vi "RPi HMI Loop.vi"() -> ()   [LabVIEW 2019]
uses:
  Controls/RPi HMI Mode.ctl
  Controls/HMI Global Mode.ctl
panel:
  in  "Power Relay":T1
  in  "Manual\nCMD":dbl[](array[numeric])=[0.0, 0.0, 0.0, 0.0, 0.0, 0.0] min=0.0 max=100.0 step=0.1 format="%#.2f"
  in  "Power Supply Cmd (V):":dbl min=0.0 max=20.0 format="%#.2f"
  in  "PressureCMD":dbl caption="Pressure Cmd (kPa):" min=0.0 max=825.0 format="%#.2f"
  in  "pb.Run Profile":bool
  in  "Tank 1 Setpoint":dbl caption="deg C"
  in  "Tank 2 Setpoint":dbl caption="deg C"
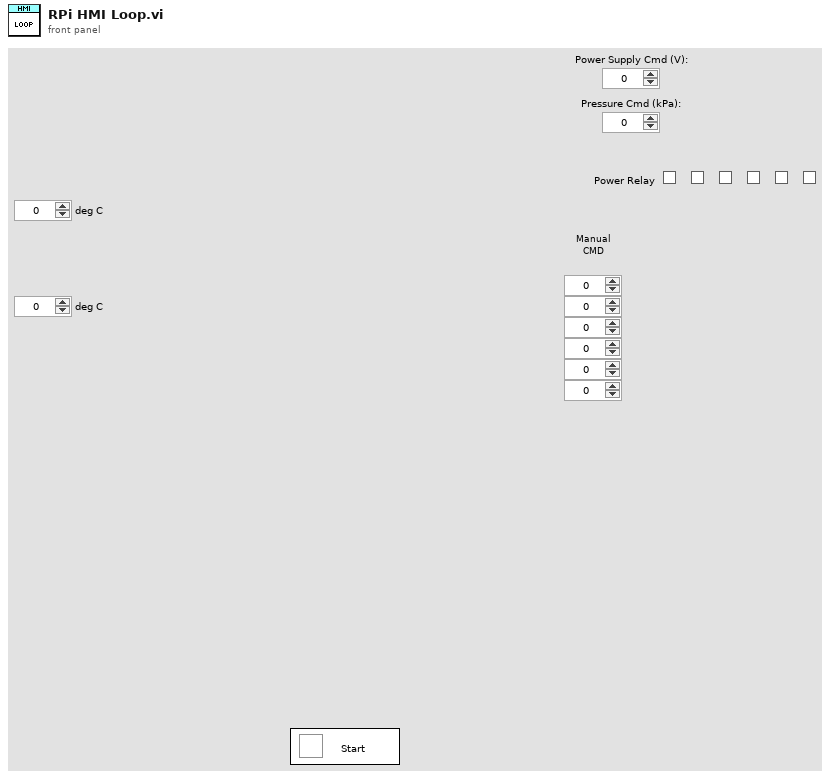
[diagram p1: front panel]
types:
  T1 = cluster{"Pump 1":bool, "Pump 2":bool, "Pump 3":bool, "Pump 4":bool, "Pump 5":bool, "Pump 6":bool}
  T2 = typedef "RPi HMI Mode.ctl" = enum16{"Init", "Write Data", "Read from RPi", "Write to RPi", "Read HMI Cluster"}
  T3 = typedef "HMI Cluster.ctl" = cluster{"Error":errorcluster, "COM Ref":refnum<visa-resource-name>, "Pump Data":T4, "Tank Data":cluster{"PS Actual (V):":dbl, "Temp1":dbl, "Temp2":dbl}, "Power Relays":cluster{"Pump 1":bool, "Pump 2":bool, "Pump 3":bool, "Pump 4":bool, "Pump 5":bool, "Pump 6":bool}, "Pump CMDs":dbl[], "HMI Header":T5, "Tank CMDs":T6, "HMI Tog Buttons":T7, "In Test":bool, "HMI Command":bool, "HMI Mom Buttons":T8, "Controller Config":T9, "Alarm":bool, "Alarm Message 1":string, "Alarm Message 2":string, "Recording":bool, "Serial Numbers":string[], "Pumps Present":bool[]}
  T4 = typedef "Pump Data.ctl" = cluster{"Voltages":dbl[], "PumpCurrent":dbl[], "Speed":dbl[], "ControllerCurrent":dbl[], "Pressure":dbl[], "Flow":dbl[], "Elapsed Time (Display)":dbl[], "Avg Pressure":dbl, "Avg Speed":dbl, "Elapsed Time":dbl[], "Diagnostic":dbl[]}
  T5 = typedef "HMI Header.ctl" = cluster{"Line 1":string, "Line 2":string, "Line 3":string, "Line 4":string}
  T6 = typedef "Tank CMDs.ctl" = cluster{"PS CMD":dbl, "Press CMD":dbl, "Temp 1 CMD":dbl, "Temp 2 CMD":dbl, "AO2 CMD":dbl}
  T7 = typedef "HMI Tog Buttons.ctl" = cluster{"Start Test":bool, "Toggle Spare 1":bool, "Toggle Spare 2":bool, "Toggle Spare 3":bool, "Toggle Spare 4":bool, "Toggle Spare 5":bool}
  T8 = typedef "HMI Mom Buttons.ctl" = cluster{"Stop":bool, "Reset Timers":bool, "Log Fuel Change":bool, "Alarm Dismiss":bool}
  T9 = typedef "Controller Config.ctl" = cluster{"Controller Name":T10, "CommSeg":i32, "PWM?":bool, "Frequency":i32, "Low Command":dbl, "High Command":dbl, "Stop Command":dbl, "Command Step":dbl, "Solenoid Stop?":bool, "Controller?":bool, "Invert PWM":bool, "Flange Mount Ctrl":bool, "Diagnostic Mode":T11}
  T10 = typedef "Controller Names.ctl" = enum16{"Kuhnke", "Helbako BLDC", "Conti", "Hella BLDC OL PWM", "Hella BLDC Turbine OL PWM", "Hella BLDC Pressure", "Helbako (old)", "TI PWM", "PSA", "Hella Gas", "Hella Diesel", "8 Comm", "10 Comm", "8 Comm Hella", "10 Comm Hella", "8 Comm Omron", "10 Comm Omron", "8 Comm Nissan", "10 Comm Nissan", "8 Comm Hella (for FCA)", "Mazda BLDC", "CMFB"}
  T11 = typedef "Diagnostic Mode.ctl" = enum16{"None", "PSA", "CMFB"}
  T12 = typedef "HMI Global Mode.ctl" = enum16{"Read", "Write Cluster", "Reset Cmd"}
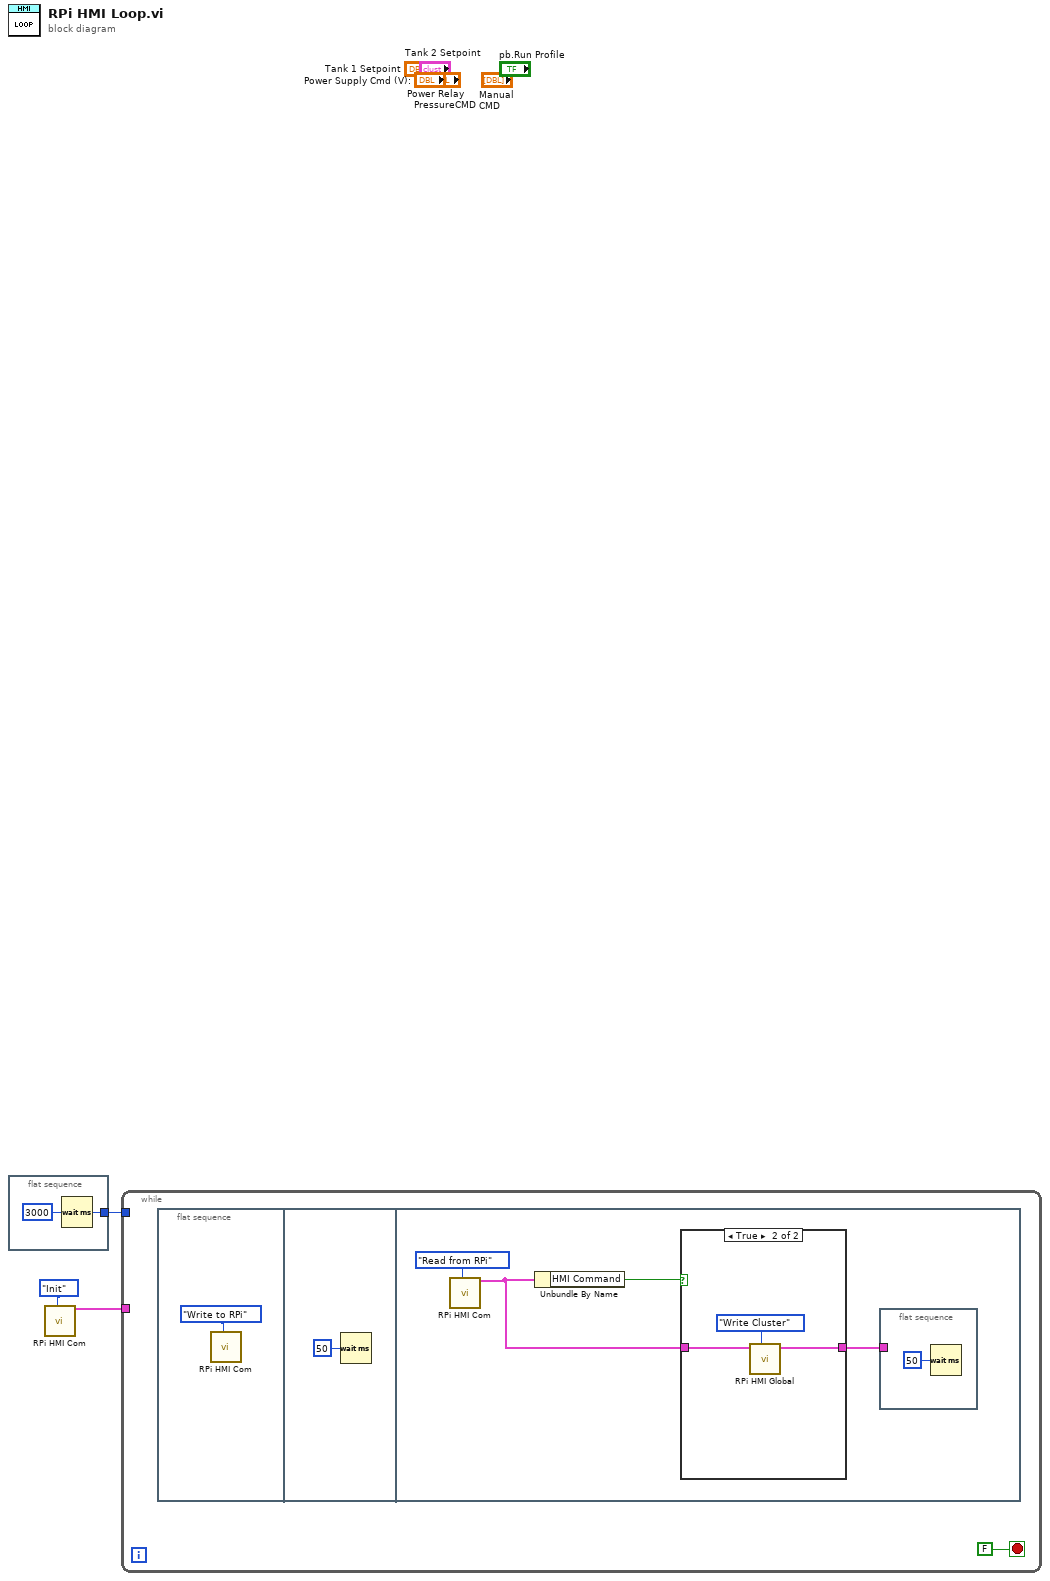
[diagram p0: block diagram]
diagram:
  n1 = flat-sequence {
    tunnel: [w4] -> w3
    frame #0 {
      n2 = Wait (ms)(milliseconds to wait=u32 3000) -> (millisecond timer value=w4:u32)
    }
  }
  n3 = call "RPi HMI Com.vi"("RPi HMI Mode"=RPi_HMI_Mode."Init") -> ("HMI Cluster"=w2:T3)  [unwired: 18 in]
  n4 = while {
    tunnel: w2 -> [_]
    tunnel: w3 -> [_]
    stop <- FALSE stop-if-true
    n5 = flat-sequence {
      frame #0 {
        n6 = call "RPi HMI Com.vi"("RPi HMI Mode"=RPi_HMI_Mode."Write to RPi") -> ()  [unwired: 18 in, 1 out]
      }
      frame #1 {
        n7 = Wait (ms)(milliseconds to wait=u32 50) -> ()  [unwired: 1 out]
      }
      frame #2 {
        n8 = call "RPi HMI Com.vi"("RPi HMI Mode"=RPi_HMI_Mode."Read from RPi") -> ("HMI Cluster"=w10:T3)  [unwired: 18 in]
        n9 = Unbundle By Name(w10) -> ("HMI Command"=w11:bool)
        n10 = case shown="True" w11 {
          tunnel: w10 -> [w14 w17]
          tunnel: [w14 w15] -> w9
          frame False {
          }
          frame True {
            n11 = call "RPi HMI Global.vi"("Mode"=HMI_Global_Mode."Write Cluster", "HMI Cluster"=w17) -> ("HMI Cluster OUT"=w15:T3)  [unwired: 9 in]
          }
        }
        n12 = flat-sequence {
          tunnel: w9 -> [_]
          frame #0 {
            n13 = Wait (ms)(milliseconds to wait=u32 50) -> ()  [unwired: 1 out]
          }
        }
      }
    }
  }
